vi "Inventory-SearchFinGoods.vi"(7 "Part Number to Search For":string, 8 "error in (no error)":errorcluster, 11 "Inventory Listbox":refnum<vi>) -> (0 "error out":errorcluster)   [LabVIEW 2013, in "ERP-Inventory.lvclass"]
uses:
  ERP-Inventory.lvclass
  <vilib>/Utility/error.llb/Error Cluster From Error Code.vi
  <vilib>/ErrorRing/Error Ring.xnode
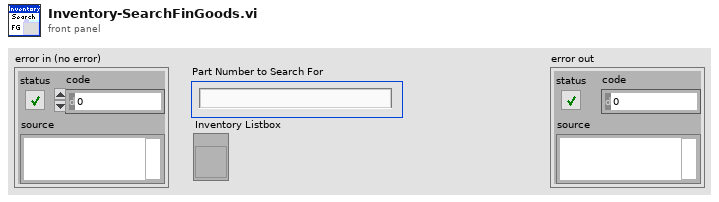
[diagram p1: front panel]
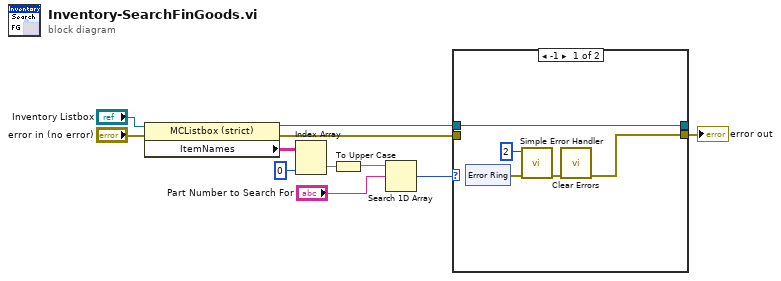
[diagram p0: block diagram]
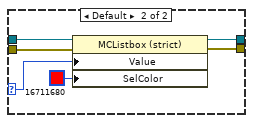
[diagram p2: hidden frame]
diagram:
  n1 = property class="MCListbox (strict)"(reference="Inventory Listbox", error in="error in (no error)") -> (reference out=w2:refnum<vi>, error out=w3:errorcluster, "ItemNames"=w10:string[][])
  n2 = Index Array(array=w10, index (col)=0 ("disabled index (col)")) -> (element=w8:string[])  [unwired: 1 in]
  n3 = To Upper Case(1:w8) -> (0:w7:string[])
  n4 = Search 1D Array(1D array=w7, element="Part Number to Search For") -> (index of element=w4:i32)  [unwired: 1 in]
  n5 = case shown="-1" w4 {
    selector: w4 -> [_ w25]
    tunnel: w3 -> [_ w27]
    tunnel: w2 -> [w14 w26]
    tunnel: [w12 w23] -> w1
    tunnel: [w14 w22] -> _
    frame -1 {
      n6 = xnode "Error Ring"() -> ("error out"=w15:errorcluster)
      n7 = call <vilib>:"Simple Error Handler.vi"("error code (no error:0)"=2, "error in (no error)"=w15) -> ("error out"=w13:errorcluster)  [unwired: 3 in, 4 out]
      n8 = call <vilib>:"Clear Errors.vi"("error in (no error)"=w13) -> ("error out"=w12:errorcluster)  [unwired: 6 in]
    }
    frame Default {
      n9 = property class="MCListbox (strict)"(reference=w26, error in=w27, "Value"=w25, "SelColor"=u32 16711680) -> (reference out=w22:refnum<vi>, error out=w23:errorcluster)
    }
  }
  "error out" <- w1
